vi "Dashboard Read-Write.vi"() -> ()   [LabVIEW 2012]
uses:
  Robot Global Data.vi
panel:
  out "Loop Time 3":u32(graph)
  out "Loop Time 2":u32(graph)
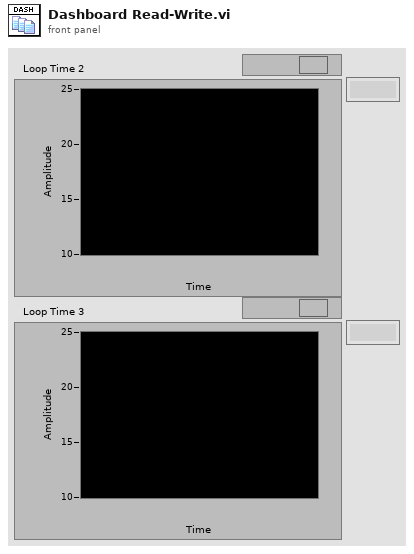
[diagram p1: front panel]
types:
  T1 = typedef "WPI_DigitalInputDevRef.ctl" = cluster{"DevStatus":errorcluster, "DIO Channel":T2, "Digital Module":T3}
  T2 = typedef "FPGA_DIOChannel.ctl" = enum8{"DIO 1", "DIO 2", "DIO 3", "DIO 4", "DIO 5", "DIO 6", "DIO 7", "DIO 8", "DIO 9", "DIO 10", "DIO 11", "DIO 12", "DIO 13", "DIO 14", "Invalid"}
  T3 = typedef "FPGA_TypedefDigitalModule.ctl" = enum16{"Digital Module 1", "Digital Module 2"}
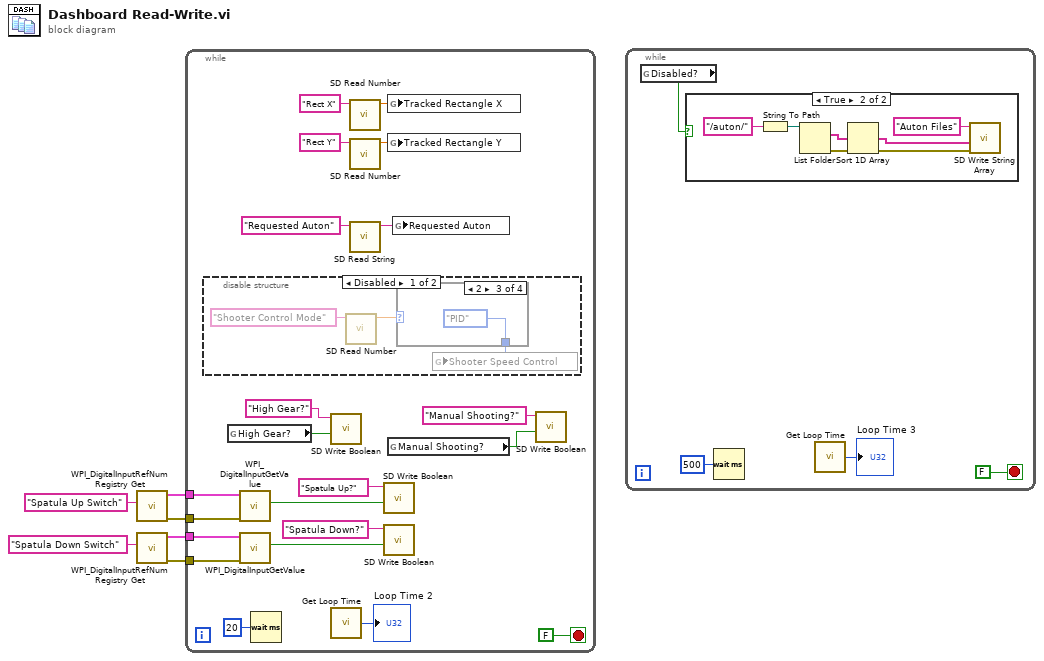
[diagram p0: block diagram]
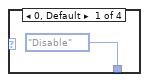
[diagram p3: hidden frame]
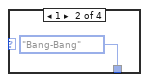
[diagram p4: hidden frame]
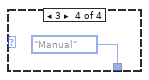
[diagram p5: hidden frame]
diagram:
  n1 = call <vilib>:"WPI_DigitalInputRefNum Registry Get.vi"("refnum name"="Spatula Up Switch") -> ("error out"=w4:errorcluster, "DigitalInputDevRef"=w5:T1)  [unwired: 9 in]
  n2 = call <vilib>:"WPI_DigitalInputRefNum Registry Get.vi"("refnum name"="Spatula Down Switch") -> ("error out"=w3:errorcluster, "DigitalInputDevRef"=w2:T1)  [unwired: 9 in]
  n3 = while {
    tunnel: w5 -> [w15]
    tunnel: w4 -> [w14]
    tunnel: w2 -> [w8]
    tunnel: w3 -> [w9]
    stop <- FALSE stop-if-true
    n4 = disable-structure shown="Disabled" {
      frame Disabled {
        n5 = call <vilib>:"SD Read Number.vi"("Name"="Shooter Control Mode") -> ("Numeric"=w29:dbl)  [unwired: 8 in, 2 out]
        n6 = case shown="2" w29 {
          tunnel: [enum16{"Disable", "Bang-Bang", "PID", "Manual"}."Disable" ("Shooter Speed Control") enum16{"Disable", "Bang-Bang", "PID", "Manual"}."Bang-Bang" ("Shooter Speed Control") enum16{"Disable", "Bang-Bang", "PID", "Manual"}."PID" ("Shooter Speed Control") enum16{"Disable", "Bang-Bang", "PID", "Manual"}."Manual" ("Shooter Speed Control")] -> w28
          frame 0, Default {
          }
          frame 1 {
          }
          frame 2 {
          }
          frame 3 {
          }
        }
        n7 = global write "Robot Global Data.vi" "Shooter Speed Control"(w28) -> ()
      }
      frame Enabled {
      }
    }
    n8 = global read "Robot Global Data.vi" "High Gear?"() -> (w18:bool)
    n9 = call <vilib>:"WPI_DigitalInputGetValue.vi"("error in (no error)"=w14, "DigitalInputDevRef"=w15) -> ("Value"=w12:bool)  [unwired: 7 in, 2 out]
    n10 = call <vilib>:"WPI_DigitalInputGetValue.vi"("error in (no error)"=w9, "DigitalInputDevRef"=w8) -> ("Value"=w11:bool)  [unwired: 7 in, 2 out]
    n11 = Wait (ms)(milliseconds to wait=u32 20) -> ()  [unwired: 1 out]
    n12 = call <vilib>:"SD Write Boolean.vi"("Boolean"=w18, "Name"="High Gear?") -> ()  [unwired: 8 in, 2 out]
    n13 = call "Get Loop Time.vi"() -> ("Loop Time"=→"Loop Time 2":u32)  [unwired: 1 in]
    n14 = call <vilib>:"SD Read Number.vi"("Name"="Rect X") -> ("Numeric"=w26:dbl)  [unwired: 8 in, 2 out]
    n15 = call <vilib>:"SD Read Number.vi"("Name"="Rect Y") -> ("Numeric"=w25:dbl)  [unwired: 8 in, 2 out]
    n16 = call <vilib>:"SD Read String.vi"("Name"="Requested Auton") -> ("String"=w20:string)  [unwired: 8 in, 2 out]
    n17 = call <vilib>:"SD Write Boolean.vi"("Boolean"=w12, "Name"="Spatula Up?") -> ()  [unwired: 8 in, 2 out]
    n18 = call <vilib>:"SD Write Boolean.vi"("Boolean"=w11, "Name"="Spatula Down?") -> ()  [unwired: 8 in, 2 out]
    n19 = global write "Robot Global Data.vi" "Tracked Rectangle X"(w26) -> ()
    n20 = global write "Robot Global Data.vi" "Tracked Rectangle Y"(w25) -> ()
    n21 = global read "Robot Global Data.vi" "Manual Shooting?"() -> (w7:bool)
    n22 = global write "Robot Global Data.vi" "Requested Auton"(w20) -> ()
    n23 = call <vilib>:"SD Write Boolean.vi"("Boolean"=w7, "Name"="Manual Shooting?") -> ()  [unwired: 8 in, 2 out]
  }
  n24 = while {
    stop <- FALSE stop-if-true
    n25 = global read "Robot Global Data.vi" "Disabled?"() -> (w36:bool)
    n26 = case shown="True" w36 {
      frame False {
      }
      frame True {
        n27 = String To Path(string="/auton/") -> (path=w44:path)
        n28 = List Folder(path=w44) -> (filenames=w40:string[], error out=w42:errorcluster)  [unwired: 1 in, 4 out]
        n29 = Sort 1D Array(array=w40) -> (sorted array=w39:string[])
        n30 = call <vilib>:"SD Write String Array.vi"("error in"=w42, "String Array"=w39, "Name"="Auton Files") -> ()  [unwired: 7 in, 2 out]
      }
    }
    n31 = Wait (ms)(milliseconds to wait=u32 500) -> ()  [unwired: 1 out]
    n32 = call "Get Loop Time.vi"() -> ("Loop Time"=→"Loop Time 3":u32)  [unwired: 1 in]
  }
